vi "Set Mode.vi"(0 "object in":refnum<class "HPS-17000-PowerModule.lvclass">, 5 "mode":string, 11 "Error In":errorcluster) -> (4 "object out":refnum<class "HPS-17000-PowerModule.lvclass">, 15 "Error Out":errorcluster)   [LabVIEW 2023, in "HPS-17000-PowerModule.lvlib" / "HPS-17000-PowerModule.lvclass"]
uses:
  HPS-17000-PowerModule.lvclass
  Mode.ctl
  <instrlib>/HPS-17000/Client Facing Datatypes/Range.ctl
  <instrlib>/HPS-17000/Client Facing Datatypes/Mode.ctl
  <instrlib>/HPS-17000/Internal/Set Mode Multi.vi
  HPS-17000-PowerModule.lvclass/HPS-17000-PowerModule.ctl
  <instrlib>/HPS-17000/HPS-17000.lvclass
panel:
  in  "MODE":T1 items=["CONSTANT CURRENT (I)", "CONSTANT VOLTAGE (V+R)", "FIXED SOURCE (V_VCC_R)", "INTERNAL RECIRCULATION (V_VCC_IINT)"]
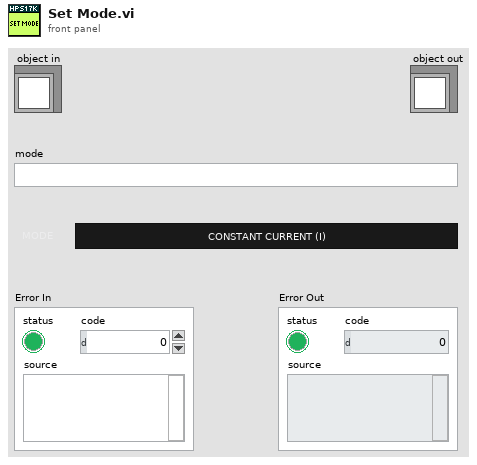
[diagram p1: front panel]
types:
  T1 = typedef "HPS-17000-PowerModule.lvlib/HPS-17000-PowerModule.lvclass/Mode.ctl" = u16
  T2 = typedef "HPS-17000-PowerModule.lvlib/HPS-17000-PowerModule.lvclass/ObjectAttributes.ctl" = cluster{"JSON Config Path":path, "Configuration":T3, "GM ID":string, "HPS17000 Refs":refnum<class "HPS-17000.lvclass">[], "connected":bool, "reserved":bool, "events":T5, "nibatterycycler_grpc_Setpoint":T6, "last timestamp":i64, "mode":T1, "range":T7, "measurement array":T8[], "measurement stream":bool, "setpoint stream":bool}
  T3 = typedef "HPS-17000-PowerModule.lvlib/HPS-17000-PowerModule.lvclass/Configuration.ctl" = cluster{"TSN NIC IP Address":string, "HPS17000 IP Addresses":string[], "HPS Topology":enum16{"SINGLE", "MULTI"}, "Setpoint Stream Config":T4, "Measurement Array Size":i32}
  T4 = typedef "Cycler.lvclass/Setpoint Stream Basic Config.ctl" = cluster{"local address":string, "receiver port":u16}
  T5 = typedef "HPS-17000.lvclass/Multi-Cycler Events.ctl" = cluster{"heartbeats events":refnum<user-event>[], "faults events":refnum<user-event>[], "network sync event":refnum<user-event>[], "setpoint status event":refnum<user-event>[]}
  T6 = typedef "NI_BC_client.lvlib/nibatterycycler_grpc_Setpoint.ctl" = cluster{"voltage":sgl, "current":sgl, "min_power":sgl, "max_power":sgl, "resistance":sgl}
  T7 = typedef "PowerModuleInterface.lvlibp/PowerModuleInterface.lvclass/Range.ctl" = cluster{"Current Max (A)":dbl, "Current Min (A)":dbl, "Voltage Max (V)":dbl, "Voltage Min (V)":dbl}
  T8 = typedef "PowerModuleInterface.lvlibp/PowerModuleInterface.lvclass/Measurements.ctl" = cluster{"measured voltage (V)":dbl, "measured current (A)":dbl, "setpoint voltage (V)":dbl, "setpoint current (A)":dbl, "timestamp":dbl}
  T9 = typedef "LVStringsAndValuesArrayTypeDef_U16.ctl" = cluster{"String":string, "Value":u16}[]
  T10 = typedef "HPS-17000.lvclass/Range.ctl" = u8
  T11 = typedef "HPS-17000.lvclass/Mode.ctl" = u8
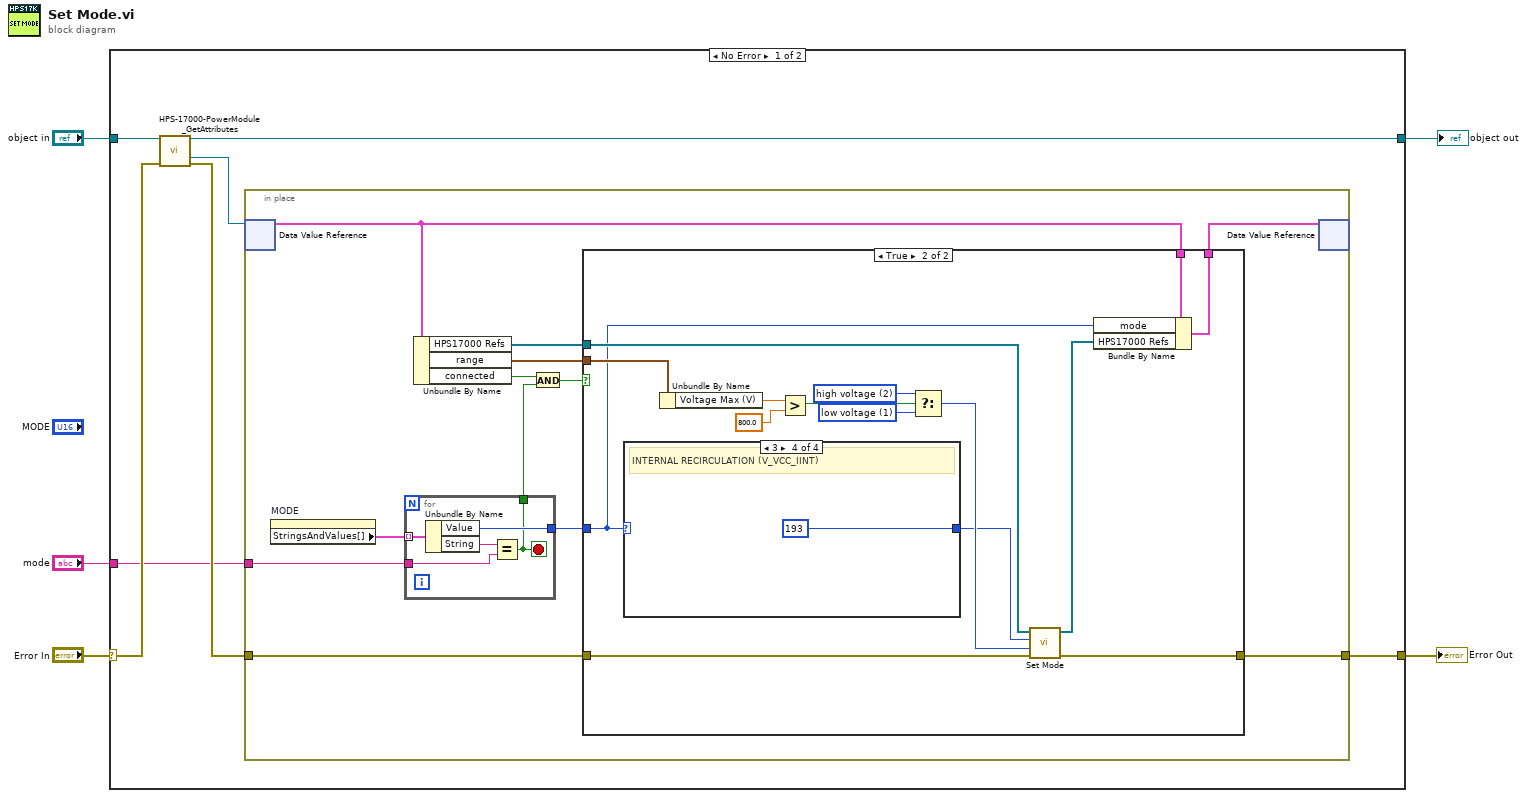
[diagram p0: block diagram]
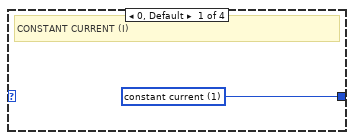
[diagram p3: hidden frame]
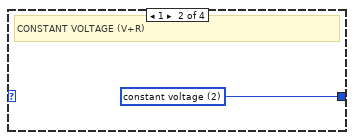
[diagram p4: hidden frame]
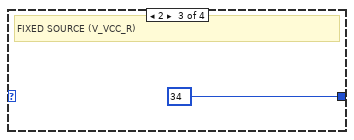
[diagram p5: hidden frame]
diagram:
  n1 = case shown="No Error" "Error In" {
    selector: "Error In" -> [w11 w51]
    tunnel: "object in" -> [w12 w52]
    tunnel: [w6 w52] -> w4
    tunnel: [w8 w51] -> w3
    tunnel: "mode" -> [w7 _]
    frame No Error {
      n2 = call "HPS-17000-PowerModule_GetAttributes.vi"("reference in"=w12, "Error In"=w11) -> ("reference out"=w6:refnum<class "HPS-17000-PowerModule.lvclass">, "DataRef"=w10:refnum<data-value>, "Error Out"=w9:errorcluster)  [unwired: 10 in, 1 out]
      n3 = in-place {
        in-place-border: w9 -> [w17]
        in-place-border: [w22] -> w8
        in-place-border: w7 -> [w18]
        n4 = in-place-dvr #1(w10) -> (w23:T2)  [unwired: 1 out]
        n5 = property on="MODE" class="Ring (strict)"() -> ("StringsAndValues[]"=w19:T9)  [unwired: 2 in, 2 out]
        n6 = for {
          tunnel: w19 -> [w29] mode=indexing
          tunnel: w18 -> [w27]
          tunnel: [w26] -> w16
          tunnel: [w25] -> w13
          stop <- w25 stop-if-true
          n7 = Unbundle By Name(w29) -> ("Value"=w26:u16, "String"=w28:string)
          n8 = Equal?(x=w28, y=w27) -> (x = y?=w25:bool)
        }
        n9 = Unbundle By Name(w23) -> ("HPS17000 Refs"=w21:refnum<class "HPS-17000.lvclass">[], "range"=w20:T7, "connected"=w15:bool)
        n10 = And(x=w15, y=w13) -> (x .and. y?=w14:bool)
        n11 = case shown="True" w14 {
          tunnel: [w31 w46] -> w24
          tunnel: w23 -> [w31 w45]
          tunnel: w17 -> [w30 w44]
          tunnel: [w30 w42] -> w22
          tunnel: w21 -> [_ w41]
          tunnel: w20 -> [_ w37]
          tunnel: w16 -> [_ w33]
          frame False {
          }
          frame True {
            w39 = T10 1 items=["low voltage"=1, "high voltage"=2] ("range")
            w40 = T10 2 items=["low voltage"=1, "high voltage"=2] ("range")
            n12 = case shown="3" w33 {
              tunnel: [w47 w48 u8 34 u8 193] -> w32
              frame 0, Default {
                w47 = T11 1 items=["constant current"=1, "constant voltage"=2, "internal recirculation"=193] ("mode")
                # "CONSTANT CURRENT (I)"
              }
              frame 1 {
                w48 = T11 2 items=["constant current"=1, "constant voltage"=2, "internal recirculation"=193] ("mode")
                # "CONSTANT VOLTAGE (V+R)"
              }
              frame 2 {
                # "FIXED SOURCE (V_VCC_R)"
              }
              frame 3 {
                # "INTERNAL RECIRCULATION (V_VCC_IINT)"
              }
            }
            n13 = Unbundle By Name(w37) -> ("Voltage Max (V)"=w36:dbl)
            n14 = Greater?(x=w36, y=800.0) -> (0:w34:bool)
            n15 = Select(t=w40, s=w34, f=w39) -> (s? t:f=w38:T10)
            n16 = call-poly <instrlib>:"Set Mode.vi"("error in"=w44, "range"=w38, "mode"=w32, "cycler refs in"=w41) -> ("error out"=w42:errorcluster, "cycler refs out"=w43:refnum<class "HPS-17000.lvclass">[])  [unwired: 6 in]
            n17 = Bundle By Name(cluster=w45, "mode"=w33, "HPS17000 Refs"=w43) -> (w46:T2)
          }
        }
        n18 = in-place-dvr #1(w24) -> ()  [unwired: 2 out]
      }
    }
    frame Error {
    }
  }
  "Error Out" <- w3
  "object out" <- w4
